vi "Save CSV.vi"(8 "error in":errorcluster, 10 "CSV Data":string[][](array[string]), 11 "TDMS File":path) -> (0 "error out":errorcluster)   [LabVIEW 2022 SP3, in "CSV Export.lvlib" / "CSV Export.lvclass"]
uses:
  CSV Export.lvclass
  CSV Export.lvclass/CSV Export.ctl
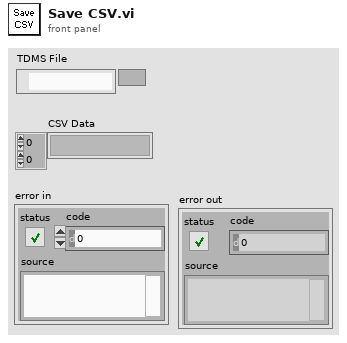
[diagram p1: front panel]
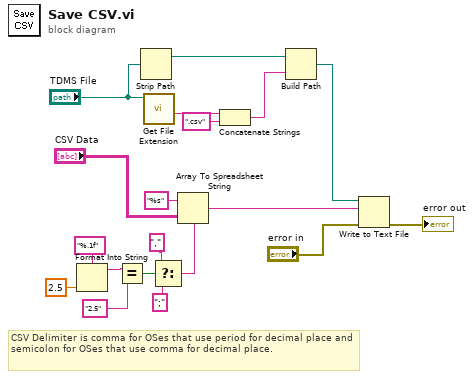
[diagram p0: block diagram]
diagram:
  # "CSV Delimiter is comma for OSes that use period for decimal place and semicolon for OSes that use comma for decimal place."
  n1 = Format Into String(format string="%.1f", 2.5 ("input 1")) -> (resulting string=w11:string)  [unwired: 2 in, 1 out]
  n2 = Equal?(x=w11, y="2.5") -> (x = y?=w13:bool)
  n3 = Strip Path(path="TDMS File") -> (stripped path=w6:path)  [unwired: 1 out]
  n4 = call <vilib>:"Get File Extension.vi"("file"="TDMS File") -> ("filename without extension"=w8:string)  [unwired: 6 in, 4 out]
  n5 = Select(t=",", s=w13, f=";") -> (s? t:f=w17:string)
  n6 = Array To Spreadsheet String(delimiter (Tab)=w17, array="CSV Data", 3:"%s" ("format string")) -> (spreadsheet string=w19:string)
  n7 = Concatenate Strings(w8, ".csv" ("string")) -> (w5:string)
  n8 = Build Path(base path=w6, name or relative path=w5) -> (appended path=w4:path)
  n9 = Write to Text File(file (use dialog)=w4, text=w19, error in="error in") -> (error out=→"error out":errorcluster)  [unwired: 1 in, 2 out]
